vi "分析仪.vi"(6 "超时":u32=10000 caption="超时（10秒）", 9 "波特率":u32=19200 caption="波特率(9600)", 10 "指令输入（不需要自己算校验码）":string="\u0001\u0003\u0000\u0000\u0000\u0001", 11 "串口":refnum<visa-resource-name>="COM5" caption="VISA资源名称") -> (2 "通讯":bool)   [LabVIEW 2015]
uses:
  <vilib>/Instr/_visa.llb/VISA Configure Serial Port (Instr).vi
panel:
  out "Out":string
  out "*(类型 *) &x":sgl
  out "子字符串":string
  out "读取缓冲区":string
  out "完整发送的数据帧(带上校验码）":string
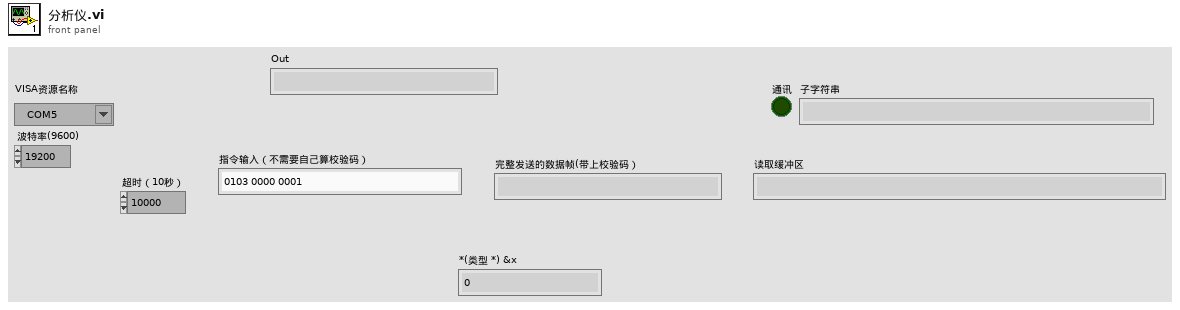
[diagram p1: front panel]
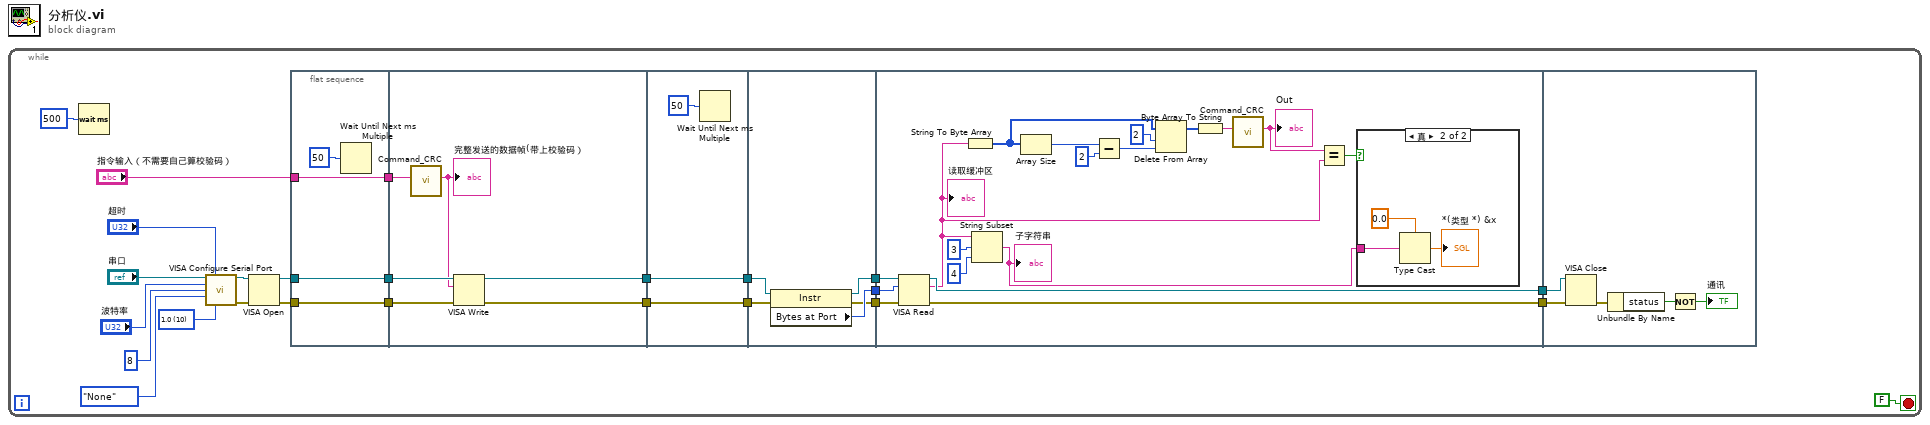
[diagram p0: block diagram]
diagram:
  n1 = while {
    stop <- FALSE stop-if-true
    w4 = u16 10 items=["1.0"=10, "1.5"=15, "2.0"=20] ("停止位")
    n2 = Wait (ms)(milliseconds to wait=u32 500 ("等待时间（毫秒）")) -> ()  [unwired: 1 out]
    n3 = call-poly "VISA Configure Serial Port"("VISA resource name"="串口", "timeout (10sec)"="超时", "baud rate (9600)"="波特率", "data bits (8)"=u16 8 ("数据位"), "parity (0:none)"=enum16{"None", "Odd", "Even", "Mark", "Space"}."None" ("奇偶校验"), "stop bits (10: 1 bit)"=w4) -> ("VISA resource name out"=w13:refnum<visa-resource-name>, "error out"=w12:errorcluster)  [unwired: 8 in]
    n4 = VISA Open(error in (no error)=w12, VISA resource name=w13) -> (VISA resource name=w9:refnum<visa-resource-name>, error out=w10:errorcluster)  [unwired: 3 in]
    n5 = flat-sequence {
      tunnel: "指令输入（不需要自己算校验码）" -> [w27]
      tunnel: w10 -> [w28]
      tunnel: w9 -> [w29]
      tunnel: [w29] -> w25
      tunnel: [w28] -> w24
      tunnel: [w27] -> w23
      tunnel: [w35] -> w22
      tunnel: [w34] -> w21
      tunnel: w25 -> [w33]
      tunnel: w24 -> [w32]
      tunnel: w23 -> [w30]
      tunnel: w22 -> [w38]
      tunnel: [w38] -> w20
      tunnel: w21 -> [w37]
      tunnel: [w37] -> w19
      tunnel: w20 -> [w41]
      tunnel: w19 -> [w43]
      tunnel: [w39] -> w18
      tunnel: [w40] -> w17
      tunnel: [w42] -> w16
      tunnel: w18 -> [w61]
      tunnel: w17 -> [w60]
      tunnel: w16 -> [w57]
      tunnel: [w59] -> w15
      tunnel: [w58] -> w14
      tunnel: w15 -> [w69]
      tunnel: w14 -> [w68]
      frame #0 {
        n6 = Wait Until Next ms Multiple(millisecond multiple=u32 50 ("毫秒倍数")) -> ()  [unwired: 1 out]
      }
      frame #1 {
        n7 = call "Command_CRC.vi"("In"=w30) -> ("Out"=w31:string)  [unwired: 9 in, 1 out]
        "完整发送的数据帧(带上校验码）" <- w31
        n8 = VISA Write(VISA resource name=w33, write buffer=w31, error in (no error)=w32) -> (VISA resource name out=w35:refnum<visa-resource-name>, error out=w34:errorcluster)  [unwired: 1 out]
      }
      frame #2 {
        n9 = Wait Until Next ms Multiple(millisecond multiple=u32 50 ("毫秒倍数")) -> ()  [unwired: 1 out]
      }
      frame #3 {
        n10 = property class="Instr"(reference=w41, error in=w43) -> (reference out=w39:refnum<visa-resource-name>, error out=w40:errorcluster, "Bytes at Port"=w42:u32)
      }
      frame #4 {
        n11 = VISA Read(VISA resource name=w61, byte count=w57, error in (no error)=w60) -> (VISA resource name out=w59:refnum<visa-resource-name>, read buffer=w44:string, error out=w58:errorcluster)  [unwired: 1 out]
        "读取缓冲区" <- w44
        n12 = String To Byte Array(string=w44) -> (unsigned byte array=w54:u8[])
        n13 = String Subset(string=w44, offset (0)=3 ("偏移量(0)"), length (rest)=4 ("长度（剩余）")) -> (substring=w46:string)
        "子字符串" <- w46
        n14 = Array Size(array=w54) -> (size(s)=w53:i32)
        n15 = Subtract(x=w53, y=2) -> (x-y=w51:i32)
        n16 = Delete From Array(array=w54, length=2 ("长度"), index=w51) -> (array with subset deleted=w49:u8[])  [unwired: 1 out]
        n17 = Byte Array To String(unsigned byte array=w49) -> (string=w48:string)
        n18 = call "Command_CRC.vi"("In"=w48) -> ("Out"=w47:string)  [unwired: 9 in, 1 out]
        "Out" <- w47
        n19 = Equal?(x=w47, y=w44) -> (x = y?=w45:bool)
        n20 = case shown="真" w45 {
          tunnel: w46 -> [_ w62]
          frame False {
          }
          frame True {
            n21 = Type Cast(type=sgl 0.0, x=w62) -> (*(type *) &x=→"*(类型 *) &x":sgl)
          }
        }
      }
      frame #5 {
        n22 = VISA Close(VISA resource name=w69, error in (no error)=w68) -> (error out=w67:errorcluster)
        n23 = Unbundle By Name(w67) -> ("status"=w66:bool)
        n24 = Not(x=w66) -> (.not. x?=→"通讯":bool)
      }
    }
  }
